vi "tcs_issueCommand_filterChangeRequest.vi"(8 "error in (no error)":errorcluster, 11 "command_filterChangeRequest_Ctl":T1) -> (0 "error out":errorcluster, 2 "function return":i32, 3 "command_filterChangeRequest_Ctl out":T1)   [LabVIEW 2016, in "SALLV_tcs.lvlib"]
doc: "int tcs_shm_issueCommand_filterChangeRequestLV(tcs_command_filterChangeRequestLV *command_filterChangeRequest_Ctl );"
uses:
  SALLV_tcs.lvlib
  DataTypes/command_filterChangeRequest.ctl
  SALLV_tcs.so
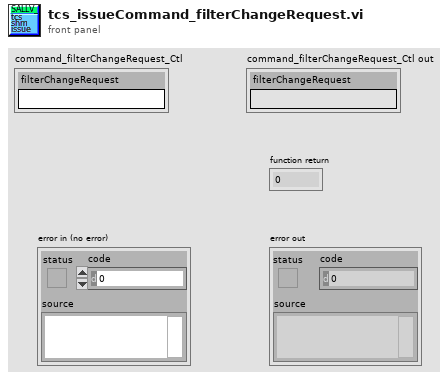
[diagram p1: front panel]
types:
  T1 = typedef "SALLV_tcs.lvlib/command_filterChangeRequest.ctl" = cluster{"filterChangeRequest":string}
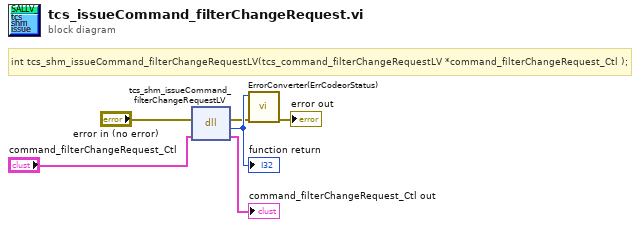
[diagram p0: block diagram]
diagram:
  # "int tcs_shm_issueCommand_filterChangeRequestLV(tcs_command_filterChangeRequestLV *command_filterChangeRequest_Ctl );"
  n1 = dll-call lib="home/andres/Desktop/SALLV_tcs/SALLV_tcs.*" fn="tcs_shm_issueCommand_filterChangeRequestLV"(error in="error in (no error)", "command_filterChangeRequest_Ctl"="command_filterChangeRequest_Ctl") -> (error out=w2:errorcluster, w6:i32, "command_filterChangeRequest_Ctl"=→"command_filterChangeRequest_Ctl out":T1)  [unwired: 2 in, 1 out]
  "function return" <- w6
  n2 = call "ErrorConverter(ErrCodeorStatus).vi"("error in (no error)"=w2, "error code"=w6) -> ("error out"=→"error out":errorcluster)  [unwired: 9 in]
